vi "FTW-JSON-Object-GetElement-Object.vi"(0 "JSON":refnum<class "FTW-Container.lvclass">, 5 "Key":string, 7 "Default Value":string, 9 "Consume Value":bool, 11 "error in":errorcluster) -> (4 "JSON out":refnum<class "FTW-Container.lvclass">, 6 "JSON Element Type":T1, 8 "Value":refnum<class "FTW-Container.lvclass">, 10 "Found":bool, 15 "error out":errorcluster)   [LabVIEW 2015]
uses:
  container/FTW-Container.lvclass
  FTW-JSON-Type.ctl
panel:
  # "Inputs"
  # "Outputs"
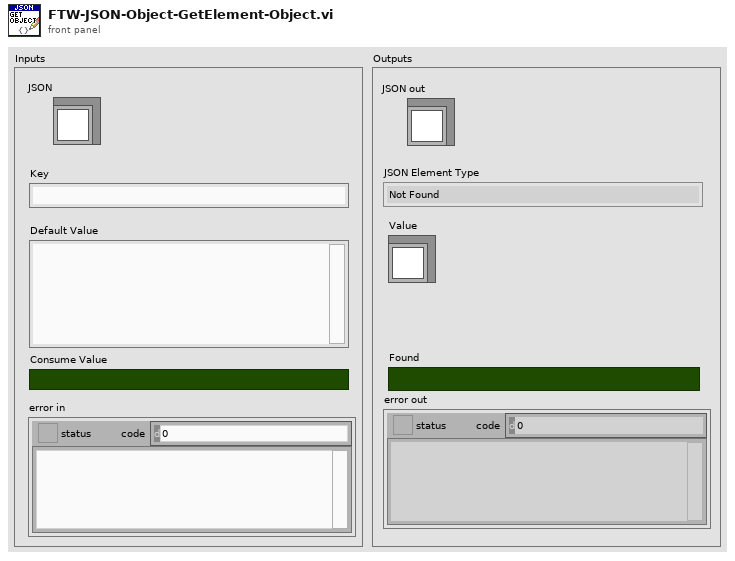
[diagram p1: front panel]
types:
  T1 = typedef "FTW-JSON-Type.ctl" = enum8{"Not Found", "Object", "Array", "String", "Number", "Boolean", "null"}
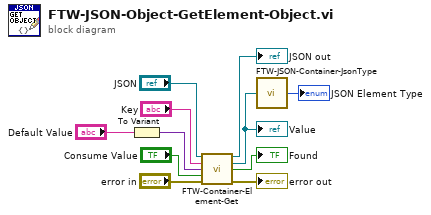
[diagram p0: block diagram]
diagram:
  n1 = To Variant(anything="Default Value") -> (Variant=w11:variant)
  n2 = call "FTW-Container-Element-Get.vi"("FTW-Container In"="JSON", "Element Name"="Key", "Default Value"=w11, "Delete?"="Consume Value", "error in"="error in") -> ("FTW-Container Out"=→"JSON out":refnum<class "FTW-Container.lvclass">, "Element Out"=w2:refnum<class "FTW-Container.lvclass">, "Found"=→"Found":bool, "error out"=→"error out":errorcluster)  [unwired: 7 in]
  "Value" <- w2
  n3 = call "FTW-JSON-Container-JsonType.vi"("Container"=w2) -> ("JSON Element Type"=→"JSON Element Type":T1)  [unwired: 14 in]
